vi "GPIB_APEXOSA_Spectrum_Scan.vi"() -> ()   [LabVIEW 2020]
panel:
  in  "APEX Folder":string="D:\\SaveFiles\\"
  out "Errors":errorcluster={"Status"=FALSE, "Code"=1073676293, "Source"="VISA Read in APEX-sweep_start.vi->OSA Spectrum I Scan.vi"}
  in  "Sweep Stop Frequency":dbl[unit]=193445690000000.0 min=170000000000000.0 max=200000000000000.0 format="%.6p"
  in  "Sweep Start Frequency":dbl[unit]=193383298000000.0 min=170000000000000.0 max=200000000000000.0 format="%.6p"
  out "Measurement Progress":u32(slide)=200 max=11 scale=0.0..200.0
  in  "Number Steps Current":i32=20 min=1
  in  "APEX VISA":refnum<visa-resource-name>="APEX_OSA"
  # "Present Measurement"
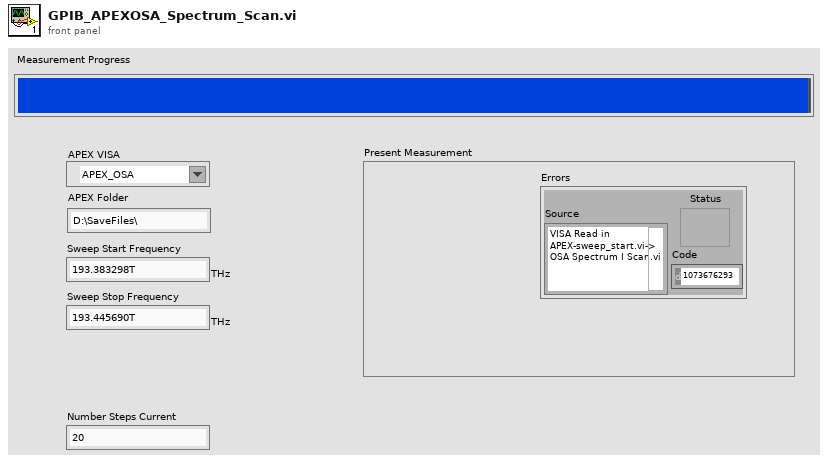
[diagram p1: front panel]
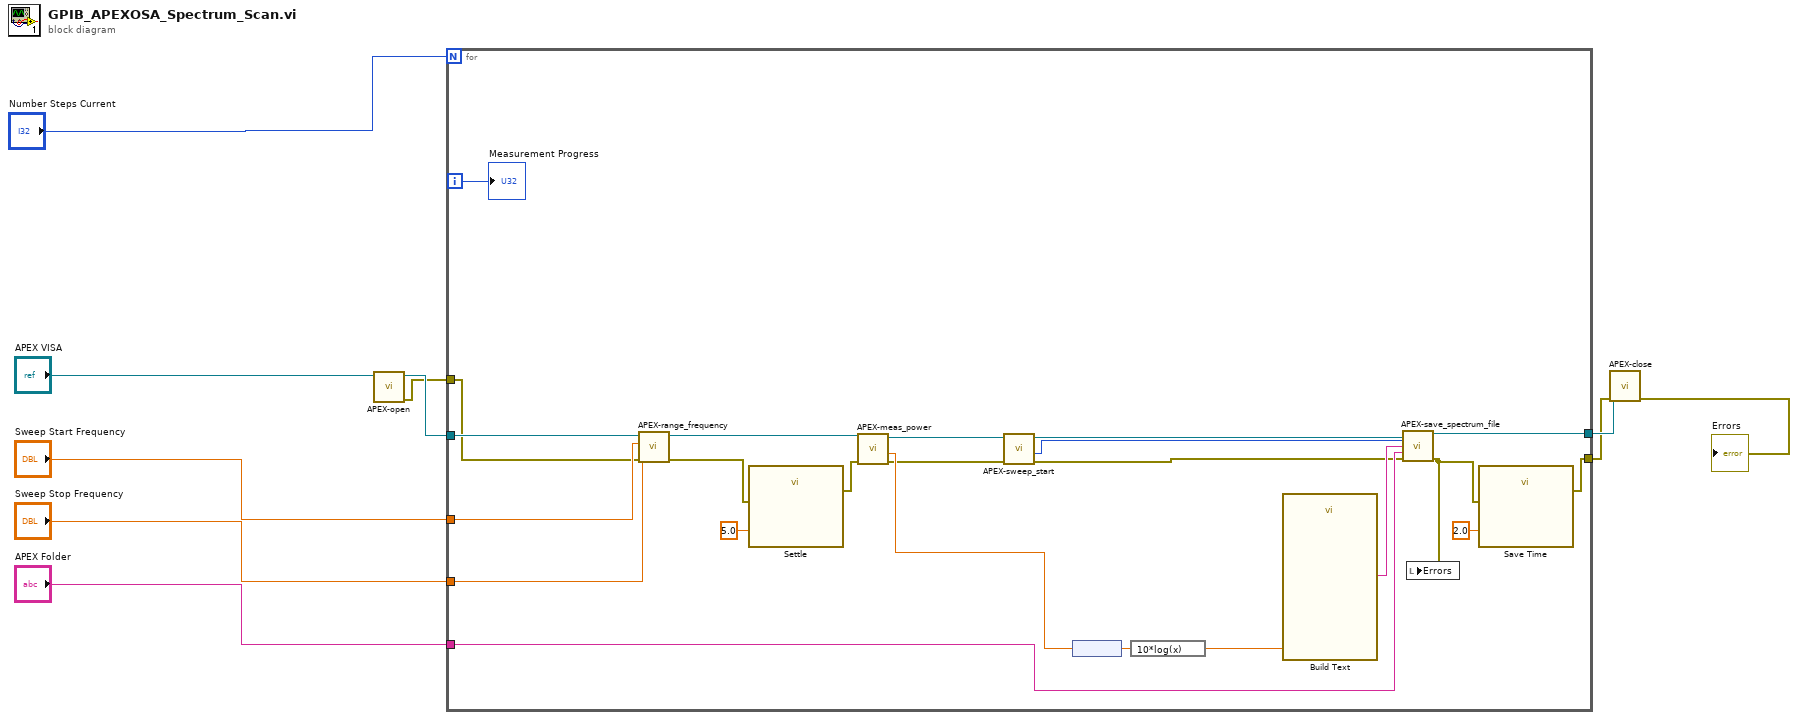
[diagram p0: block diagram]
diagram:
  n1 = call "APEX-open.vi"("VISA resource input"="APEX VISA") -> ("error out"=w8:errorcluster, "VISA resource output"=w9:refnum<visa-resource-name>)  [unwired: 8 in, 1 out]
  n2 = for {
    N: "Number Steps Current" -> [_]
    tunnel: w9 -> [w31]
    tunnel: w8 -> [w14]
    tunnel: "Sweep Start Frequency" -> [w28]
    tunnel: "Sweep Stop Frequency" -> [w29]
    tunnel: [w13] -> w5
    tunnel: [w24] -> w4
    tunnel: "APEX Folder" -> [w27]
    i -> [w33]
    n3 = call "APEX-range_frequency.vi"("error in (no error)"=w14, "Sweep Stop Frequency"=w29, "Sweep Start Frequency"=w28, "VISA resource input"=w31) -> ("error out"=w16:errorcluster, "VISA resource output"=w17:refnum<visa-resource-name>)  [unwired: 6 in]
    n4 = call "Settle"("error in (no error)"=w16, "Delay Time (s)"=5.0) -> ("error out"=w20:errorcluster)  [unwired: 9 in]
    n5 = call "APEX-meas_power.vi"("error in (no error)"=w20, "VISA resource input"=w17) -> ("error out"=w15:errorcluster, "Optical Power 1"=w18:dbl[unit], "VISA resource output"=w21:refnum<visa-resource-name>)  [unwired: 7 in]
    n6 = call "APEX-sweep_start.vi"("error in (no error)"=w15, "VISA resource input"=w21) -> ("error out"=w12:errorcluster, "Trace Number"=w26:i32, "VISA resource output"=w30:refnum<visa-resource-name>)  [unwired: 7 in]
    n7 = node(w18) -> (w19:dbl)
    n8 = expression code="10*log(x)"(w19) -> (w11:dbl)
    n9 = call "Build Text"("Optical Power"=w11) -> ("Result"=w22:string)  [unwired: 13 in, 1 out]
    n10 = call "APEX-save_spectrum_file.vi"("VISA resource input"=w30, "Trace Number"=w26, "File Name"=w22, "File Path"=w27, "error in (no error)"=w12) -> ("VISA resource output"=w13:refnum<visa-resource-name>, "error out"=w25:errorcluster)  [unwired: 9 in]
    n11 = local write "Errors"(w25) -> ()
    n12 = call "Save Time"("error in (no error)"=w25, "Delay Time (s)"=2.0) -> ("error out"=w24:errorcluster)  [unwired: 9 in]
    "Measurement Progress" <- w33
  }
  n13 = call "APEX-close.vi"("error in (no error)"=w4, "VISA resource input"=w5) -> ("error out"=→"Errors":errorcluster)  [unwired: 9 in]
